vi "ANALOG Command to Data.vi"(11 "Teszt cluster":T1) -> (1 "Min":dbl, 2 "Max":dbl, 3 "Variable Name":string)   [LabVIEW 2014]
uses:
  Teszt/Teszt.ctl
  Teszt/Command.ctl
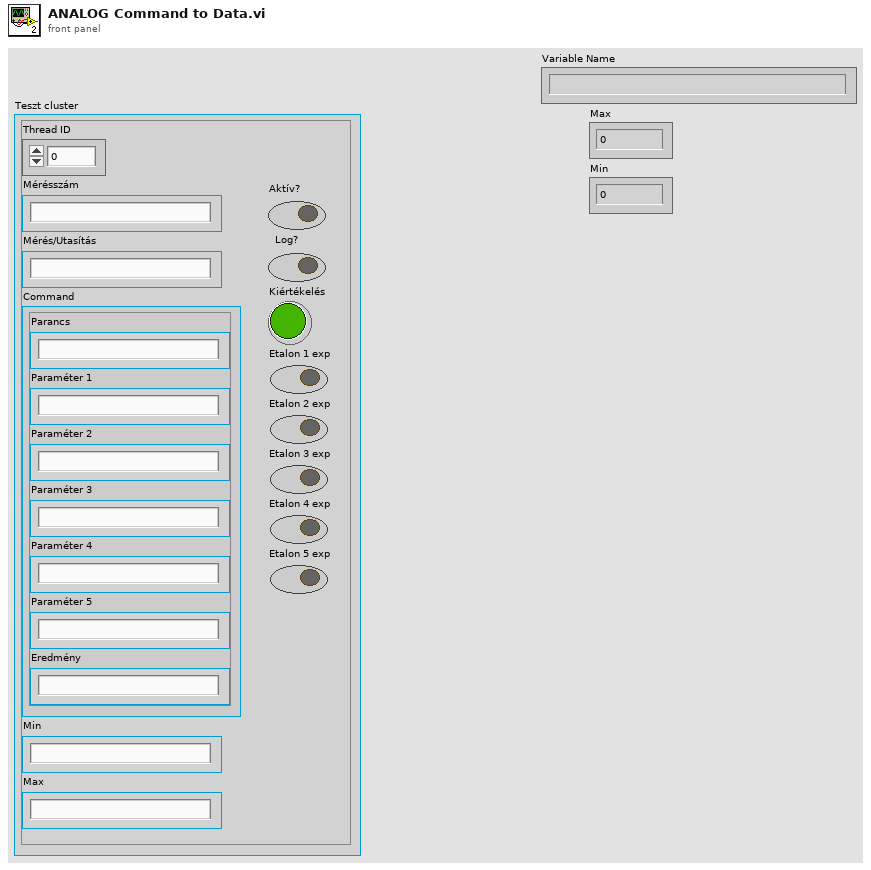
[diagram p1: front panel]
types:
  T1 = typedef "Teszt.ctl" = cluster{"Thread ID":dbl, "Mérésszám":string, "Mérés/Utasítás":string, "Command":T2, "Min":string, "Max":string, "Aktív?":bool, "Log?":bool, "Kiértékelés":bool, "Etalon 1 exp":bool, "Etalon 2 exp":bool, "Etalon 3 exp":bool, "Etalon 4 exp":bool, "Etalon 5 exp":bool}
  T2 = typedef "Command.ctl" = cluster{"Parancs":string, "Paraméter 1":string, "Paraméter 2":string, "Paraméter 3":string, "Paraméter 4":string, "Paraméter 5":string, "Eredmény":string}
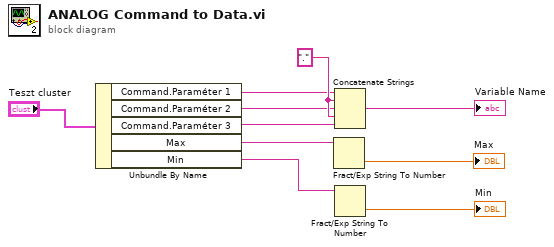
[diagram p0: block diagram]
diagram:
  w9 = "."
  n1 = Unbundle By Name("Teszt cluster") -> ("Command.Paraméter 1"=w6:string, "Command.Paraméter 2"=w7:string, "Command.Paraméter 3"=w8:string, "Max"=w4:string, "Min"=w3:string)
  n2 = Fract/Exp String To Number(string=w4) -> (number=→"Max":dbl)  [unwired: 3 in, 1 out]
  n3 = Concatenate Strings(w6, w9, w7, w9, w8) -> (→"Variable Name":string)
  n4 = Fract/Exp String To Number(string=w3) -> (number=→"Min":dbl)  [unwired: 3 in, 1 out]
